vi "Secure-Release Region.vi"(7 "Action":enum16{"Secure", "Release"}(ring), 8 "error in (no error)":errorcluster, 10 "Control In":T1={"I-O.lvclass"=refnum, "Gantry"=refnum, "Dispenser"="COM1"}, 11 "Carrier Tray in":refnum<class "Assembly Tray.lvclass">) -> (0 "error out":errorcluster, 1 "Position":i32, 2 "Control Out":T1={"I-O.lvclass"=refnum, "Gantry"=refnum, "Dispenser"="COM1"}, 3 "Carrier Tray out":refnum<class "Assembly Tray.lvclass">)   [LabVIEW 2021, in "Assembly Tray.lvclass"]
uses:
  Assembly Tray.lvclass
  C:/Users/HEP/Documents/GitHub/Gantry/UCSB-Gantry-HEP-main/Classes/Workspace/Fixture.lvclass
  Controller/Controllers.ctl
  Controller/I-O/I-O.lvclass
  C:/Program Files (x86)/Aerotech/A3200/LabVIEW/2010/Bin/Aerotech.A3200.dll
  Program Files (x86)/Aerotech/A3200/LabVIEW/2010/Bin/Aerotech.A3200.dll
  Fixture.lvclass/Fixture.ctl
  Assembly Tray.lvclass/Assembly Tray.ctl
  Fixture.lvclass
  Controller/Motion/Motion.lvclass
  Controller/Controller.lvclass
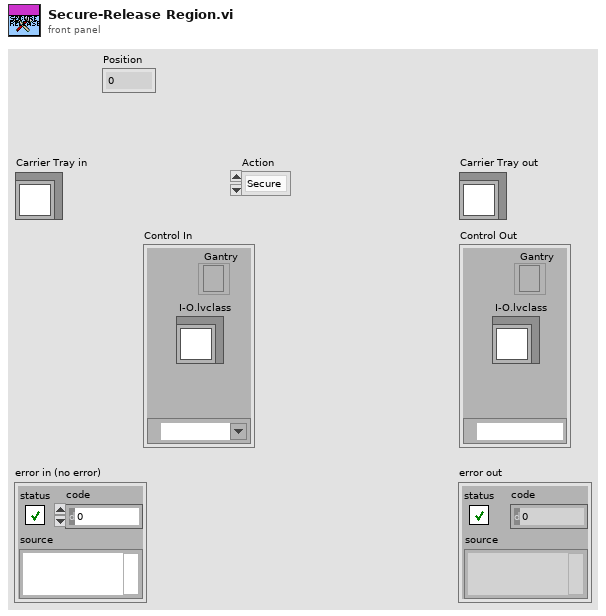
[diagram p1: front panel]
types:
  T1 = typedef "Controller.lvclass/Controllers.ctl" = cluster{"I-O.lvclass":refnum<class "I-O.lvclass">, "Gantry":refnum<k24>, "Dispenser":refnum<visa-resource-name>}
  T2 = typedef "I-O.lvclass/Pin Map.ctl" = cluster{"Region Valves":i32[], "Extra Valves":dbl[][][], "Tool Primary Valve":i32, "Tool Secondary Valve":i32, "Region Sensors":i32[], "Extra Sensors":dbl[][][], "Tool Primary Sensor":dbl, "Tool Secondary Sensor":dbl, "Compression Sensor":dbl, "5V":i32, "Dispenser Sensor":dbl}
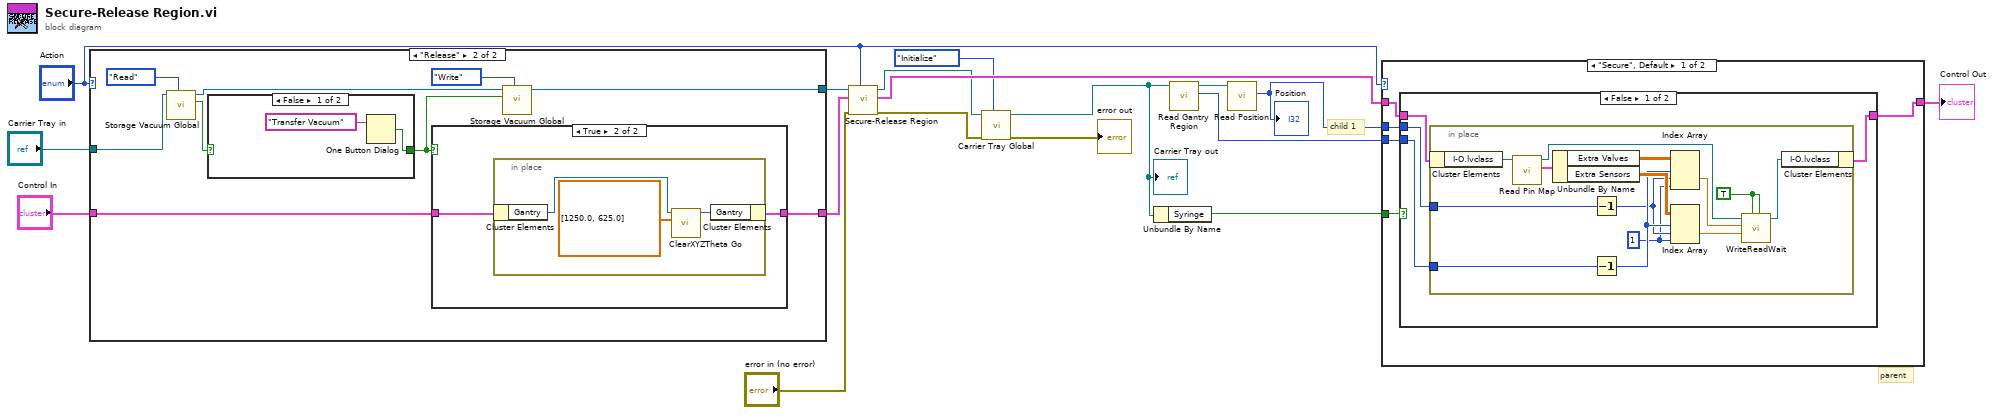
[diagram p0: block diagram]
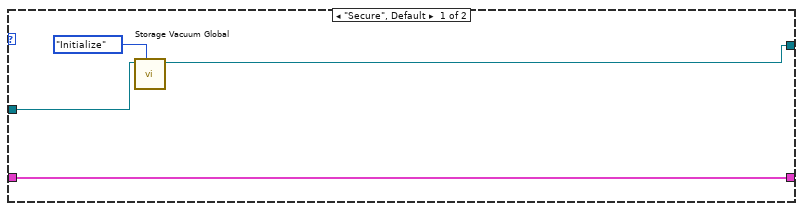
[diagram p4: hidden frame]
diagram:
  # "child 1"
  # "parent"
  n1 = case shown="\"Release\"" "Action" {
    tunnel: [w20 w26] -> w15
    tunnel: "Carrier Tray in" -> [w19 w25]
    tunnel: "Control In" -> [w18 w23]
    tunnel: [w18 w22] -> w1
    frame "Secure", Default {
      n2 = call "Storage Vacuum Global.vi"("Action"=enum16{"Initialize", "Read", "Write"}."Initialize", "Carrier Tray.lvclass"=w19) -> ("Carrier Tray.lvclass 2"=w20:refnum<class "Assembly Tray.lvclass">)  [unwired: 7 in, 2 out]
    }
    frame "Release" {
      n3 = call "Storage Vacuum Global.vi"("Action"=enum16{"Initialize", "Read", "Write"}."Read", "Carrier Tray.lvclass"=w25) -> ("Read"=w30:bool, "Carrier Tray.lvclass 2"=w27:refnum<class "Assembly Tray.lvclass">)  [unwired: 7 in, 1 out]
      n4 = case shown="False" w30 {
        selector: w30 -> [_ w39]
        tunnel: [w37 w39] -> w24
        frame False {
          n5 = One Button Dialog(message="Transfer Vacuum") -> (true=w37:bool)  [unwired: 1 in]
        }
        frame True {
        }
      }
      n6 = case shown="True" w24 {
        tunnel: w23 -> [w31 w33]
        tunnel: [w31 w32] -> w22
        frame False {
        }
        frame True {
          n7 = in-place {
            n8 = in-place-cluster #1(w33) -> ("Gantry"=w35:refnum<k24>)
            n9 = call "ClearXYZTheta Go.vi"("XYZTheta In"=dbl[] [1250.0, 625.0], "Gantry In"=w35) -> ("Gantry Out"=w34:refnum<k24>)  [unwired: 7 in, 2 out]
            n10 = in-place-cluster #1("Gantry"=w34) -> (w32:T1)
          }
        }
      }
      n11 = call "Storage Vacuum Global.vi"("Action"=enum16{"Initialize", "Read", "Write"}."Write", "Write"=w24, "Carrier Tray.lvclass"=w27) -> ("Carrier Tray.lvclass 2"=w26:refnum<class "Assembly Tray.lvclass">)  [unwired: 6 in, 2 out]
    }
  }
  n12 = call-parent "Secure-Release Region.vi"("Action"="Action", "error in (no error)"="error in (no error)", "Control In"=w1, "Fixture in"=w15) -> ("error out"=w5:errorcluster, "Control Out"=w13:T1, "Fixture out"=w8:refnum<class "Assembly Tray.lvclass">)  [unwired: 4 in, 1 out]
  n13 = call "Carrier Tray Global.vi"("Action"=enum16{"Initialize", "Read", "Write"}."Initialize", "error in (no error)"=w5, "Carrier Tray.lvclass"=w8) -> ("error out"=→"error out":errorcluster, "Carrier Tray.lvclass 2"=w7:refnum<class "Assembly Tray.lvclass">)  [unwired: 6 in, 1 out]
  "Carrier Tray out" <- w7
  n14 = Unbundle By Name(w7) -> ("Syringe"=w14:bool)
  n15 = call "Read Gantry Region.vi"("Fixture in"=w7) -> ("Gantry Region"=w11:i32, "Fixture out"=w12:refnum<class "Assembly Tray.lvclass">)  [unwired: 8 in, 1 out]
  n16 = call "Read Position.vi"("Fixture in"=w12) -> ("Position"=w3:i32)  [unwired: 8 in, 2 out]
  "Position" <- w3
  n17 = case shown="\"Secure\", Default" "Action" {
    tunnel: w14 -> [w44 _]
    tunnel: w13 -> [w43 w64]
    tunnel: w11 -> [w42 _]
    tunnel: w3 -> [w41 _]
    tunnel: [w40 w64] -> w10
    frame "Secure", Default {
      n18 = case shown="False" w44 {
        tunnel: w43 -> [w48 w63]
        tunnel: w42 -> [w47 _]
        tunnel: w41 -> [w46 _]
        tunnel: [w45 w63] -> w40
        frame False {
          n19 = in-place {
            in-place-border: w47 -> [w56]
            in-place-border: w46 -> [w54]
            w52 = 1
            w58 = TRUE
            n20 = in-place-cluster #2(w48) -> ("I-O.lvclass"=w62:refnum<class "I-O.lvclass">)
            n21 = call-dynamic "Read Pin Map.vi"("I-O in"=w62) -> ("Pin Map 2"=w61:T2, "I-O out"=w59:refnum<class "I-O.lvclass">)  [unwired: 8 in, 1 out]
            n22 = Unbundle By Name(w61) -> ("Extra Valves"=w49:dbl[][][], "Extra Sensors"=w60:dbl[][][])
            n23 = Decrement(x=w54) -> (x-1=w53:i32)
            n24 = Decrement(x=w56) -> (x-1=w55:i32)
            n25 = Index Array(array=w49, index (dim 0)=w55, index (dim 1)=w53, index (dim 2)=w52) -> (element=w51:dbl)
            n26 = Index Array(array=w60, index (dim 0)=w55, index (dim 1)=w53, index (dim 2)=w52) -> (element=w50:dbl)
            n27 = call "WriteReadWait.vi"("Read Value"=w58, "Write Value"=w58, "Read"=w50, "Write"=w51, "I-O in"=w59) -> ("I-O out"=w57:refnum<class "I-O.lvclass">)  [unwired: 5 in, 1 out]
            n28 = in-place-cluster #2("I-O.lvclass"=w57) -> (w45:T1)
          }
        }
        frame True {
        }
      }
    }
    frame "Release" {
    }
  }
  "Control Out" <- w10
